vi "Set Operating Mode.vi"(3 "error in":errorcluster, 4 "Operating Mode":bool[](array[boolean]), 5 "COM Port in":refnum<visa-resource-name>) -> (0 "error out":errorcluster, 1 "OK":bool, 2 "COM Port out":refnum<visa-resource-name>)   [LabVIEW 2013]
doc: "This command sets several operating mode states in one command.\n\nPlease refer to the \"Get operating mode\" chapter for a detailed description of the \"operating mode\" parameter."
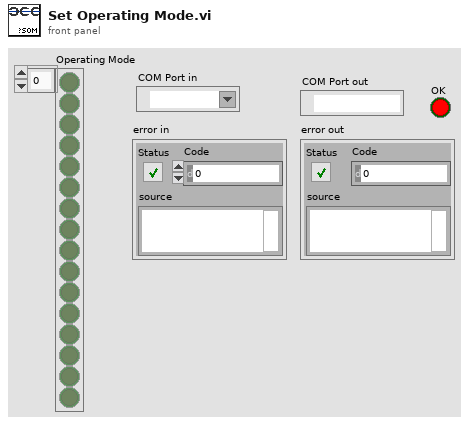
[diagram p1: front panel]
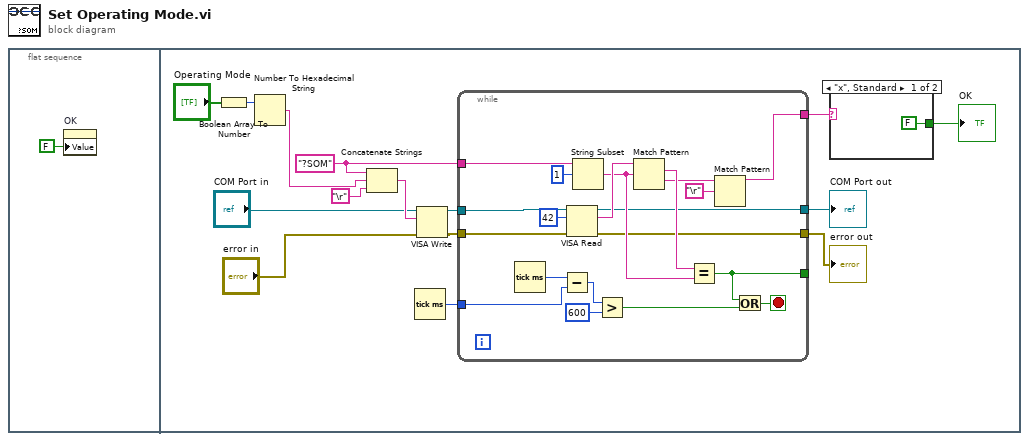
[diagram p0: block diagram]
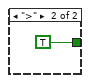
[diagram p2: hidden frame]
diagram:
  n1 = flat-sequence {
    frame #0 {
      n2 = property on="OK" class="Bool. (strikt)"("Value"=FALSE ("OK")) -> ()  [unwired: 2 in, 2 out]
    }
    frame #1 {
      w9 = "?SOM" ("Schreibpuffer")
      n3 = Boolean Array To Number(Boolean array="Operating Mode") -> (number=w4:u32)
      n4 = Number To Hexadecimal String(2:w4) -> (0:w2:string)  [unwired: 1 in]
      n5 = Concatenate Strings(w9, w2, "\r") -> (w14:string)
      n6 = Tick Count (ms)() -> (millisecond timer value=w8:u32)
      n7 = VISA Write(VISA resource name="COM Port in", write buffer=w14, error in (no error)="error in") -> (VISA resource name out=w11:refnum<visa-resource-name>, error out=w10:errorcluster)  [unwired: 1 out]
      n8 = while {
        tunnel: [w33] -> w16
        tunnel: [w32] -> w15
        tunnel: [w31] -> w7
        tunnel: [w27] -> _
        tunnel: w11 -> [w20]
        tunnel: w10 -> [w29]
        tunnel: w9 -> [w28]
        tunnel: w8 -> [w24]
        stop <- w26 stop-if-true
        n9 = Tick Count (ms)() -> (millisecond timer value=w25:u32)
        n10 = Subtract(x=w25, y=w24) -> (x-y=w23:u32)
        n11 = VISA Read(VISA resource name=w20, byte count=u32 42 ("Byte-Anzahl"), error in (no error)=w29) -> (VISA resource name out=w33:refnum<visa-resource-name>, read buffer=w37:string, error out=w32:errorcluster)  [unwired: 1 out]
        n12 = String Subset(string=w28, offset (0)=1 ("Offset (0)")) -> (substring=w34:string)  [unwired: 1 in]
        n13 = Greater?(x=w23, y=u32 600) -> (0:w21:bool)
        n14 = Match Pattern(string=w37, regular expression=w34) -> (match substring=w36:string, after substring=w30:string)  [unwired: 1 in, 2 out]
        n15 = Equal?(x=w36, y=w34) -> (x = y?=w27:bool)
        n16 = Match Pattern(string=w30, regular expression="\r") -> (before substring=w31:string)  [unwired: 1 in, 3 out]
        n17 = Or(x=w27, y=w21) -> (x .or. y?=w26:bool)
      }
      "COM Port out" <- w16
      "error out" <- w15
      n18 = case shown="\"x\", Standard" w7 {
        tunnel: [FALSE TRUE] -> w6
        frame "x", Default {
        }
        frame ">" {
        }
      }
      "OK" <- w6
    }
  }
